vi "Rotate 1D Array.vi"(2 "n":i32, 3 "array":dbl[](array[numeric]) format="%.2f") -> (1 "array (last n elements first)":dbl[](array[numeric]) format="%.2f")   [LabVIEW 2017, in "NI_AdvCtrl_continuous linear.lvlib"]
doc: "LabVIEW no longer supports this VI. You can obtain similar functionality by installing the LabVIEW Simulation Module.\n\nThis VI produces the same result as the Rotate 1D Array function in LabVIEW, however it does not allocate and deallocate memory on each call."
uses:
  <vilib>/addons/control/advanced/NI_AdvCtrl_continuous linear.lvlib
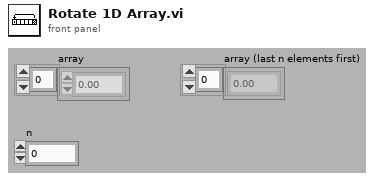
[diagram p1: front panel]
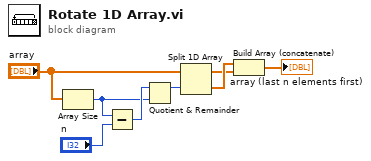
[diagram p0: block diagram]
diagram:
  n1 = Array Size(array="array") -> (size(s)=w1:i32)
  n2 = Subtract(x=w1, y="n") -> (x-y=w2:i32)
  n3 = Quotient & Remainder(x=w2, y=w1) -> (x-y*floor(x/y)=w3:i32)  [unwired: 1 out]
  n4 = Split 1D Array(array="array", index=w3) -> (first subarray=w5:dbl[], second subarray=w6:dbl[])
  n5 = Build Array (concatenate)(w6, w5) -> (→"array (last n elements first)":dbl[])
